vi "GetLinkerInfoFromFile.vi"(8 "error in (no error)":errorcluster, 10 "path in":path, 11 "CDependencyInspector in":refnum<class "CDependencyInspection.lvclass">) -> (0 "error out":errorcluster, 2 "Linker.Read Info From File":T2(array[cluster]), 3 "CDependencyInspector out":refnum<class "CDependencyInspection.lvclass">)   [LabVIEW 2020, in "DependencyInspection.lvlib" / "CDependencyInspection.lvclass"]
uses:
  CDependencyInspection.lvclass
  <vilib>/Utility/lvfile.llb/LVFileType.ctl
  <vilib>/Utility/lvfile.llb/NI_FileType.lvlib
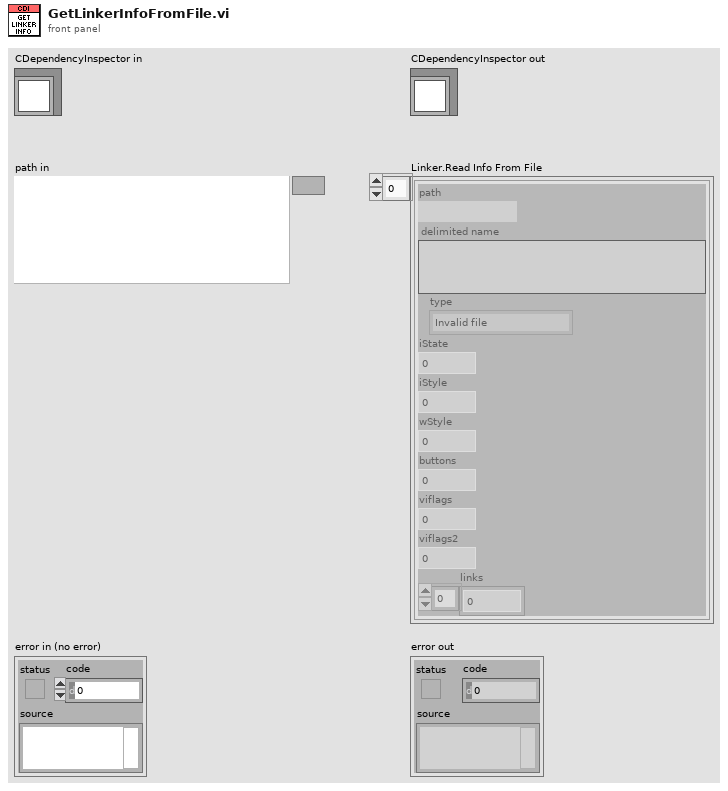
[diagram p1: front panel]
types:
  T1 = typedef "NI_FileType.lvlib/LVFileType.ctl" = enum32{"Invalid file", "Unknown type", "Instrument", "Control", "Polymorphic VI", "Project", "Library", "LVClass", "XControl", "XNode", "Shared library", ".NET assembly", "ActiveX interface", "CIN", "Run-time menu", "Palette menu", "Help file", "LLB", "XNode Edit Dependency", "Class Private Data Control", "Statechart", "MathScript .m file", "Ladder Diagram", "LVLibp", "XNode Build Dependency"}
  T2 = cluster{"path":path, "delimited name":string, "type":T1, "iState":u32, "iStyle":u16, "wStyle":u16, "buttons":u16, "viflags":u32, "viflags2":u32, "links":u32[]}[]
  T3 = cluster{"path":path, "delimited name":string, "type":T1, "iState":u32, "iStyle":u16, "wStyle":u16, "buttons":u16, "viflags":u32, "viflags2":u32, "links":u32[]}
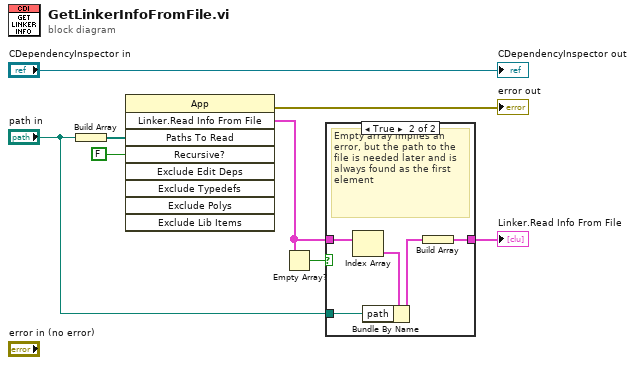
[diagram p0: block diagram]
diagram:
  n1 = Build Array("path in") -> (w7:path[])
  n2 = invoke class="App" method="Linker.Read Info From File"("Paths To Read"=w7, "Recursive?"=FALSE) -> (error out=→"error out":errorcluster, "Linker.Read Info From File"=w4:T2)  [unwired: 7 in, 7 out]
  n3 = Empty Array?(array=w4) -> (empty?=w3:bool)
  n4 = case shown="True" w3 {
    tunnel: w4 -> [w9 w14]
    tunnel: [w9 w10] -> w2
    tunnel: "path in" -> [_ w12]
    frame False {
    }
    frame True {
      # "Empty array implies an error, but the path to the file is needed later and is always found as the first element"
      n5 = Index Array(array=w14) -> (element=w13:T3)  [unwired: 1 in]
      n6 = Bundle By Name(cluster=w13, "path"=w12) -> (w11:T3)
      n7 = Build Array(w11) -> (w10:T2)
    }
  }
  "Linker.Read Info From File" <- w2
  "CDependencyInspector out" <- "CDependencyInspector in"
